vi "FipsAdjacent.vi"() -> (11 "Fips":i32[](array[numeric]))   [LabVIEW 2017] (continued)
\"Lake County, FL\"\t12069\n\"Volusia County, FL\"\t12127\t\"Marion County, FL\"\t12083\n\"Volusia County, FL\"\t12127\t\"Orange County, FL\"\t12095\n\"Volusia County, FL\"\t12127\t\"Putnam County, FL\"\t12107\n\"Volusia County, FL\"\t12127\t\"Seminole County, FL\"\t12117\n\"Volusia County, FL\"\t12127\t\"Volusia County, FL\"\t12127\n\"Wakulla County, FL\"\t12129\t\"Franklin County, FL\"\t12037\n\"Wakulla County, FL\"\t12129\t\"Jefferson County, FL\"\t12065\n\"Wakulla County, FL\"\t12129\t\"Leon County, FL\"\t12073\n\"Wakulla County, FL\"\t12129\t\"Liberty County, FL\"\t12077\n\"Wakulla County, FL\"\t12129\t\"Wakulla County, FL\"\t12129\n\"Walton County, FL\"\t12131\t\"Covington County, AL\"\t01039\n\"Walton County, FL\"\t12131\t\"Geneva County, AL\"\t01061\n\"Walton County, FL\"\t12131\t\"Bay County, FL\"\t12005\n\"Walton County, FL\"\t12131\t\"Holmes County, FL\"\t12059\n\"Walton County, FL\"\t12131\t\"Okaloosa County, FL\"\t12091\n\"Walton County, FL\"\t12131\t\"Walton County, FL\"\t12131\n\"Walton County, FL\"\t12131\t\"Washington County, FL\"\t12133\n\"Washington County, FL\"\t12133\t\"Bay County, FL\"\t12005\n\"Washington County, FL\"\t12133\t\"Holmes County, FL\"\t12059\n\"Washington County, FL\"\t12133\t\"Jackson County, FL\"\t12063\n\"Washington County, FL\"\t12133\t\"Walton County, FL\"\t12131\n\"Washington County, FL\"\t12133\t\"Washington County, FL\"\t12133\n\"Appling County, GA\"\t13001\t\"Appling County, GA\"\t13001\n\"Appling County, GA\"\t13001\t\"Bacon County, GA\"\t13005\n\"Appling County, GA\"\t13001\t\"Jeff Davis County, GA\"\t13161\n\"Appling County, GA\"\t13001\t\"Pierce County, GA\"\t13229\n\"Appling County, GA\"\t13001\t\"Tattnall County, GA\"\t13267\n\"Appling County, GA\"\t13001\t\"Toombs County, GA\"\t13279\n\"Appling County, GA\"\t13001\t\"Wayne County, GA\"\t13305\n\"Atkinson County, GA\"\t13003\t\"Atkinson County, GA\"\t13003\n\"Atkinson County, GA\"\t13003\t\"Berrien County, GA\"\t13019\n\"Atkinson County, GA\"\t13003\t\"Clinch County, GA\"\t13065\n\"Atkinson County, GA\"\t13003\t\"Coffee County, GA\"\t13069\n\"Atkinson County, GA\"\t13003\t\"Lanier County, GA\"\t13173\n\"Atkinson County, GA\"\t13003\t\"Ware County, GA\"\t13299\n\"Bacon County, GA\"\t13005\t\"Appling County, GA\"\t13001\n\"Bacon County, GA\"\t13005\t\"Bacon County, GA\"\t13005\n\"Bacon County, GA\"\t13005\t\"Coffee County, GA\"\t13069\n\"Bacon County, GA\"\t13005\t\"Jeff Davis County, GA\"\t13161\n\"Bacon County, GA\"\t13005\t\"Pierce County, GA\"\t13229\n\"Bacon County, GA\"\t13005\t\"Ware County, GA\"\t13299\n\"Baker County, GA\"\t13007\t\"Baker County, GA\"\t13007\n\"Baker County, GA\"\t13007\t\"Calhoun County, GA\"\t13037\n\"Baker County, GA\"\t13007\t\"Decatur County, GA\"\t13087\n\"Baker County, GA\"\t13007\t\"Dougherty County, GA\"\t13095\n\"Baker County, GA\"\t13007\t\"Early County, GA\"\t13099\n\"Baker County, GA\"\t13007\t\"Miller County, GA\"\t13201\n\"Baker County, GA\"\t13007\t\"Mitchell County, GA\"\t13205\n\"Baldwin County, GA\"\t13009\t\"Baldwin County, GA\"\t13009\n\"Baldwin County, GA\"\t13009\t\"Hancock County, GA\"\t13141\n\"Baldwin County, GA\"\t13009\t\"Jones County, GA\"\t13169\n\"Baldwin County, GA\"\t13009\t\"Putnam County, GA\"\t13237\n\"Baldwin County, GA\"\t13009\t\"Washington County, GA\"\t13303\n\"Baldwin County, GA\"\t13009\t\"Wilkinson County, GA\"\t13319\n\"Banks County, GA\"\t13011\t\"Banks County, GA\"\t13011\n\"Banks County, GA\"\t13011\t\"Franklin County, GA\"\t13119\n\"Banks County, GA\"\t13011\t\"Habersham County, GA\"\t13137\n\"Banks County, GA\"\t13011\t\"Hall County, GA\"\t13139\n\"Banks County, GA\"\t13011\t\"Jackson County, GA\"\t13157\n\"Banks County, GA\"\t13011\t\"Madison County, GA\"\t13195\n\"Banks County, GA\"\t13011\t\"Stephens County, GA\"\t13257\n\"Barrow County, GA\"\t13013\t\"Barrow County, GA\"\t13013\n\"Barrow County, GA\"\t13013\t\"Clarke County, GA\"\t13059\n\"Barrow County, GA\"\t13013\t\"Gwinnett County, GA\"\t13135\n\"Barrow County, GA\"\t13013\t\"Hall County, GA\"\t13139\n\"Barrow County, GA\"\t13013\t\"Jackson County, GA\"\t13157\n\"Barrow County, GA\"\t13013\t\"Oconee County, GA\"\t13219\n\"Barrow County, GA\"\t13013\t\"Walton County, GA\"\t13297\n\"Bartow County, GA\"\t13015\t\"Bartow County, GA\"\t13015\n\"Bartow County, GA\"\t13015\t\"Cherokee County, GA\"\t13057\n\"Bartow County, GA\"\t13015\t\"Cobb County, GA\"\t13067\n\"Bartow County, GA\"\t13015\t\"Floyd County, GA\"\t13115\n\"Bartow County, GA\"\t13015\t\"Gordon County, GA\"\t13129\n\"Bartow County, GA\"\t13015\t\"Paulding County, GA\"\t13223\n\"Bartow County, GA\"\t13015\t\"Pickens County, GA\"\t13227\n\"Bartow County, GA\"\t13015\t\"Polk County, GA\"\t13233\n\"Ben Hill County, GA\"\t13017\t\"Ben Hill County, GA\"\t13017\n\"Ben Hill County, GA\"\t13017\t\"Coffee County, GA\"\t13069\n\"Ben Hill County, GA\"\t13017\t\"Irwin County, GA\"\t13155\n\"Ben Hill County, GA\"\t13017\t\"Telfair County, GA\"\t13271\n\"Ben Hill County, GA\"\t13017\t\"Turner County, GA\"\t13287\n\"Ben Hill County, GA\"\t13017\t\"Wilcox County, GA\"\t13315\n\"Berrien County, GA\"\t13019\t\"Atkinson County, GA\"\t13003\n\"Berrien County, GA\"\t13019\t\"Berrien County, GA\"\t13019\n\"Berrien County, GA\"\t13019\t\"Coffee County, GA\"\t13069\n\"Berrien County, GA\"\t13019\t\"Cook County, GA\"\t13075\n\"Berrien County, GA\"\t13019\t\"Irwin County, GA\"\t13155\n\"Berrien County, GA\"\t13019\t\"Lanier County, GA\"\t13173\n\"Berrien County, GA\"\t13019\t\"Lowndes County, GA\"\t13185\n\"Berrien County, GA\"\t13019\t\"Tift County, GA\"\t13277\n\"Bibb County, GA\"\t13021\t\"Bibb County, GA\"\t13021\n\"Bibb County, GA\"\t13021\t\"Crawford County, GA\"\t13079\n\"Bibb County, GA\"\t13021\t\"Houston County, GA\"\t13153\n\"Bibb County, GA\"\t13021\t\"Jones County, GA\"\t13169\n\"Bibb County, GA\"\t13021\t\"Monroe County, GA\"\t13207\n\"Bibb County, GA\"\t13021\t\"Twiggs County, GA\"\t13289\n\"Bleckley County, GA\"\t13023\t\"Bleckley County, GA\"\t13023\n\"Bleckley County, GA\"\t13023\t\"Dodge County, GA\"\t13091\n\"Bleckley County, GA\"\t13023\t\"Houston County, GA\"\t13153\n\"Bleckley County, GA\"\t13023\t\"Laurens County, GA\"\t13175\n\"Bleckley County, GA\"\t13023\t\"Pulaski County, GA\"\t13235\n\"Bleckley County, GA\"\t13023\t\"Twiggs County, GA\"\t13289\n\"Bleckley County, GA\"\t13023\t\"Wilkinson County, GA\"\t13319\n\"Brantley County, GA\"\t13025\t\"Brantley County, GA\"\t13025\n\"Brantley County, GA\"\t13025\t\"Camden County, GA\"\t13039\n\"Brantley County, GA\"\t13025\t\"Charlton County, GA\"\t13049\n\"Brantley County, GA\"\t13025\t\"Glynn County, GA\"\t13127\n\"Brantley County, GA\"\t13025\t\"Pierce County, GA\"\t13229\n\"Brantley County, GA\"\t13025\t\"Ware County, GA\"\t13299\n\"Brantley County, GA\"\t13025\t\"Wayne County, GA\"\t13305\n\"Brooks County, GA\"\t13027\t\"Hamilton County, FL\"\t12047\n\"Brooks County, GA\"\t13027\t\"Jefferson County, FL\"\t12065\n\"Brooks County, GA\"\t13027\t\"Madison County, FL\"\t12079\n\"Brooks County, GA\"\t13027\t\"Brooks County, GA\"\t13027\n\"Brooks County, GA\"\t13027\t\"Colquitt County, GA\"\t13071\n\"Brooks County, GA\"\t13027\t\"Cook County, GA\"\t13075\n\"Brooks County, GA\"\t13027\t\"Lowndes County, GA\"\t13185\n\"Brooks County, GA\"\t13027\t\"Thomas County, GA\"\t13275\n\"Bryan County, GA\"\t13029\t\"Bryan County, GA\"\t13029\n\"Bryan County, GA\"\t13029\t\"Bulloch County, GA\"\t13031\n\"Bryan County, GA\"\t13029\t\"Chatham County, GA\"\t13051\n\"Bryan County, GA\"\t13029\t\"Effingham County, GA\"\t13103\n\"Bryan County, GA\"\t13029\t\"Evans County, GA\"\t13109\n\"Bryan County, GA\"\t13029\t\"Liberty County, GA\"\t13179\n\"Bulloch County, GA\"\t13031\t\"Bryan County, GA\"\t13029\n\"Bulloch County, GA\"\t13031\t\"Bulloch County, GA\"\t13031\n\"Bulloch County, GA\"\t13031\t\"Candler County, GA\"\t13043\n\"Bulloch County, GA\"\t13031\t\"Effingham County, GA\"\t13103\n\"Bulloch County, GA\"\t13031\t\"Emanuel County, GA\"\t13107\n\"Bulloch County, GA\"\t13031\t\"Evans County, GA\"\t13109\n\"Bulloch County, GA\"\t13031\t\"Jenkins County, GA\"\t13165\n\"Bulloch County, GA\"\t13031\t\"Screven County, GA\"\t13251\n\"Burke County, GA\"\t13033\t\"Burke County, GA\"\t13033\n\"Burke County, GA\"\t13033\t\"Emanuel County, GA\"\t13107\n\"Burke County, GA\"\t13033\t\"Jefferson County, GA\"\t13163\n\"Burke County, GA\"\t13033\t\"Jenkins County, GA\"\t13165\n\"Burke County, GA\"\t13033\t\"Richmond County, GA\"\t13245\n\"Burke County, GA\"\t13033\t\"Screven County, GA\"\t13251\n\"Burke County, GA\"\t13033\t\"Aiken County, SC\"\t45003\n\"Burke County, GA\"\t13033\t\"Allendale County, SC\"\t45005\n\"Burke County, GA\"\t13033\t\"Barnwell County, SC\"\t45011\n\"Butts County, GA\"\t13035\t\"Butts County, GA\"\t13035\n\"Butts County, GA\"\t13035\t\"Henry County, GA\"\t13151\n\"Butts County, GA\"\t13035\t\"Jasper County, GA\"\t13159\n\"Butts County, GA\"\t13035\t\"Lamar County, GA\"\t13171\n\"Butts County, GA\"\t13035\t\"Monroe County, GA\"\t13207\n\"Butts County, GA\"\t13035\t\"Newton County, GA\"\t13217\n\"Butts County, GA\"\t13035\t\"Spalding County, GA\"\t13255\n\"Calhoun County, GA\"\t13037\t\"Baker County, GA\"\t13007\n\"Calhoun County, GA\"\t13037\t\"Calhoun County, GA\"\t13037\n\"Calhoun County, GA\"\t13037\t\"Clay County, GA\"\t13061\n\"Calhoun County, GA\"\t13037\t\"Dougherty County, GA\"\t13095\n\"Calhoun County, GA\"\t13037\t\"Early County, GA\"\t13099\n\"Calhoun County, GA\"\t13037\t\"Randolph County, GA\"\t13243\n\"Calhoun County, GA\"\t13037\t\"Terrell County, GA\"\t13273\n\"Camden County, GA\"\t13039\t\"Nassau County, FL\"\t12089\n\"Camden County, GA\"\t13039\t\"Brantley County, GA\"\t13025\n\"Camden County, GA\"\t13039\t\"Camden County, GA\"\t13039\n\"Camden County, GA\"\t13039\t\"Charlton County, GA\"\t13049\n\"Camden County, GA\"\t13039\t\"Glynn County, GA\"\t13127\n\"Candler County, GA\"\t13043\t\"Bulloch County, GA\"\t13031\n\"Candler County, GA\"\t13043\t\"Candler County, GA\"\t13043\n\"Candler County, GA\"\t13043\t\"Emanuel County, GA\"\t13107\n\"Candler County, GA\"\t13043\t\"Evans County, GA\"\t13109\n\"Candler County, GA\"\t13043\t\"Tattnall County, GA\"\t13267\n\"Candler County, GA\"\t13043\t\"Toombs County, GA\"\t13279\n\"Carroll County, GA\"\t13045\t\"Cleburne County, AL\"\t01029\n\"Carroll County, GA\"\t13045\t\"Randolph County, AL\"\t01111\n\"Carroll County, GA\"\t13045\t\"Carroll County, GA\"\t13045\n\"Carroll County, GA\"\t13045\t\"Coweta County, GA\"\t13077\n\"Carroll County, GA\"\t13045\t\"Douglas County, GA\"\t13097\n\"Carroll County, GA\"\t13045\t\"Fulton County, GA\"\t13121\n\"Carroll County, GA\"\t13045\t\"Haralson County, GA\"\t13143\n\"Carroll County, GA\"\t13045\t\"Heard County, GA\"\t13149\n\"Carroll County, GA\"\t13045\t\"Paulding County, GA\"\t13223\n\"Catoosa County, GA\"\t13047\t\"Catoosa County, GA\"\t13047\n\"Catoosa County, GA\"\t13047\t\"Walker County, GA\"\t13295\n\"Catoosa County, GA\"\t13047\t\"Whitfield County, GA\"\t13313\n\"Catoosa County, GA\"\t13047\t\"Hamilton County, TN\"\t47065\n\"Charlton County, GA\"\t13049\t\"Baker County, FL\"\t12003\n\"Charlton County, GA\"\t13049\t\"Nassau County, FL\"\t12089\n\"Charlton County, GA\"\t13049\t\"Brantley County, GA\"\t13025\n\"Charlton County, GA\"\t13049\t\"Camden County, GA\"\t13039\n\"Charlton County, GA\"\t13049\t\"Charlton County, GA\"\t13049\n\"Charlton County, GA\"\t13049\t\"Ware County, GA\"\t13299\n\"Chatham County, GA\"\t13051\t\"Bryan County, GA\"\t13029\n\"Chatham County, GA\"\t13051\t\"Chatham County, GA\"\t13051\n\"Chatham County, GA\"\t13051\t\"Effingham County, GA\"\t13103\n\"Chatham County, GA\"\t13051\t\"Liberty County, GA\"\t13179\n\"Chatham County, GA\"\t13051\t\"Jasper County, SC\"\t45053\n\"Chattahoochee County, GA\"\t13053\t\"Russell County, AL\"\t01113\n\"Chattahoochee County, GA\"\t13053\t\"Chattahoochee County, GA\"\t13053\n\"Chattahoochee County, GA\"\t13053\t\"Marion County, GA\"\t13197\n\"Chattahoochee County, GA\"\t13053\t\"Muscogee County, GA\"\t13215\n\"Chattahoochee County, GA\"\t13053\t\"Stewart County, GA\"\t13259\n\"Chattahoochee County, GA\"\t13053\t\"Talbot County, GA\"\t13263\n\"Chattooga County, GA\"\t13055\t\"Cherokee County, AL\"\t01019\n\"Chattooga County, GA\"\t13055\t\"DeKalb County, AL\"\t01049\n\"Chattooga County, GA\"\t13055\t\"Chattooga County, GA\"\t13055\n\"Chattooga County, GA\"\t13055\t\"Floyd County, GA\"\t13115\n\"Chattooga County, GA\"\t13055\t\"Walker County, GA\"\t13295\n\"Cherokee County, GA\"\t13057\t\"Bartow County, GA\"\t13015\n\"Cherokee County, GA\"\t13057\t\"Cherokee County, GA\"\t13057\n\"Cherokee County, GA\"\t13057\t\"Cobb County, GA\"\t13067\n\"Cherokee County, GA\"\t13057\t\"Dawson County, GA\"\t13085\n\"Cherokee County, GA\"\t13057\t\"Forsyth County, GA\"\t13117\n\"Cherokee County, GA\"\t13057\t\"Fulton County, GA\"\t13121\n\"Cherokee County, GA\"\t13057\t\"Gordon County, GA\"\t13129\n\"Cherokee County, GA\"\t13057\t\"Pickens County, GA\"\t13227\n\"Clarke County, GA\"\t13059\t\"Barrow County, GA\"\t13013\n\"Clarke County, GA\"\t13059\t\"Clarke County, GA\"\t13059\n\"Clarke County, GA\"\t13059\t\"Jackson County, GA\"\t13157\n\"Clarke County, GA\"\t13059\t\"Madison County, GA\"\t13195\n\"Clarke County, GA\"\t13059\t\"Oconee County, GA\"\t13219\n\"Clarke County, GA\"\t13059\t\"Oglethorpe County, GA\"\t13221\n\"Clay County, GA\"\t13061\t\"Barbour County, AL\"\t01005\n\"Clay County, GA\"\t13061\t\"Henry County, AL\"\t01067\n\"Clay County, GA\"\t13061\t\"Calhoun County, GA\"\t13037\n\"Clay County, GA\"\t13061\t\"Clay County, GA\"\t13061\n\"Clay County, GA\"\t13061\t\"Early County, GA\"\t13099\n\"Clay County, GA\"\t13061\t\"Quitman County, GA\"\t13239\n\"Clay County, GA\"\t13061\t\"Randolph County, GA\"\t13243\n\"Clayton County, GA\"\t13063\t\"Clayton County, GA\"\t13063\n\"Clayton County, GA\"\t13063\t\"DeKalb County, GA\"\t13089\n\"Clayton County, GA\"\t13063\t\"Fayette County, GA\"\t13113\n\"Clayton County, GA\"\t13063\t\"Fulton County, GA\"\t13121\n\"Clayton County, GA\"\t13063\t\"Henry County, GA\"\t13151\n\"Clayton County, GA\"\t13063\t\"Spalding County, GA\"\t13255\n\"Clinch County, GA\"\t13065\t\"Baker County, FL\"\t12003\n\"Clinch County, GA\"\t13065\t\"Columbia County, FL\"\t12023\n\"Clinch County, GA\"\t13065\t\"Atkinson County, GA\"\t13003\n\"Clinch County, GA\"\t13065\t\"Clinch County, GA\"\t13065\n\"Clinch County, GA\"\t13065\t\"Echols County, GA\"\t13101\n\"Clinch County, GA\"\t13065\t\"Lanier County, GA\"\t13173\n\"Clinch County, GA\"\t13065\t\"Ware County, GA\"\t13299\n\"Cobb County, GA\"\t13067\t\"Bartow County, GA\"\t13015\n\"Cobb County, GA\"\t13067\t\"Cherokee County, GA\"\t13057\n\"Cobb County, GA\"\t13067\t\"Cobb County, GA\"\t13067\n\"Cobb County, GA\"\t13067\t\"Douglas County, GA\"\t13097\n\"Cobb County, GA\"\t13067\t\"Fulton County, GA\"\t13121\n\"Cobb County, GA\"\t13067\t\"Paulding County, GA\"\t13223\n\"Coffee County, GA\"\t13069\t\"Atkinson County, GA\"\t13003\n\"Coffee County, GA\"\t13069\t\"Bacon County, GA\"\t13005\n\"Coffee County, GA\"\t13069\t\"Ben Hill County, GA\"\t13017\n\"Coffee County, GA\"\t13069\t\"Berrien County, GA\"\t13019\n\"Coffee County, GA\"\t13069\t\"Coffee County, GA\"\t13069\n\"Coffee County, GA\"\t13069\t\"Irwin County, GA\"\t13155\n\"Coffee County, GA\"\t13069\t\"Jeff Davis County, GA\"\t13161\n\"Coffee County, GA\"\t13069\t\"Telfair County, GA\"\t13271\n\"Coffee County, GA\"\t13069\t\"Ware County, GA\"\t13299\n\"Colquitt County, GA\"\t13071\t\"Brooks County, GA\"\t13027\n\"Colquitt County, GA\"\t13071\t\"Colquitt County, GA\"\t13071\n\"Colquitt County, GA\"\t13071\t\"Cook County, GA\"\t13075\n\"Colquitt County, GA\"\t13071\t\"Mitchell County, GA\"\t13205\n\"Colquitt County, GA\"\t13071\t\"Thomas County, GA\"\t13275\n\"Colquitt County, GA\"\t13071\t\"Tift County, GA\"\t13277\n\"Colquitt County, GA\"\t13071\t\"Worth County, GA\"\t13321\n\"Columbia County, GA\"\t13073\t\"Columbia County, GA\"\t13073\n\"Columbia County, GA\"\t13073\t\"Lincoln County, GA\"\t13181\n\"Columbia County, GA\"\t13073\t\"McDuffie County, GA\"\t13189\n\"Columbia County, GA\"\t13073\t\"Richmond County, GA\"\t13245\n\"Columbia County, GA\"\t13073\t\"Edgefield County, SC\"\t45037\n\"Columbia County, GA\"\t13073\t\"McCormick County, SC\"\t45065\n\"Cook County, GA\"\t13075\t\"Berrien County, GA\"\t13019\n\"Cook County, GA\"\t13075\t\"Brooks County, GA\"\t13027\n\"Cook County, GA\"\t13075\t\"Colquitt County, GA\"\t13071\n\"Cook County, GA\"\t13075\t\"Cook County, GA\"\t13075\n\"Cook County, GA\"\t13075\t\"Lowndes County, GA\"\t13185\n\"Cook County, GA\"\t13075\t\"Tift County, GA\"\t13277\n\"Coweta County, GA\"\t13077\t\"Carroll County, GA\"\t13045\n\"Coweta County, GA\"\t13077\t\"Coweta County, GA\"\t13077\n\"Coweta County, GA\"\t13077\t\"Fayette County, GA\"\t13113\n\"Coweta County, GA\"\t13077\t\"Fulton County, GA\"\t13121\n\"Coweta County, GA\"\t13077\t\"Heard County, GA\"\t13149\n\"Coweta County, GA\"\t13077\t\"Meriwether County, GA\"\t13199\n\"Coweta County, GA\"\t13077\t\"Spalding County, GA\"\t13255\n\"Coweta County, GA\"\t13077\t\"Troup County, GA\"\t13285\n\"Crawford County, GA\"\t13079\t\"Bibb County, GA\"\t13021\n\"Crawford County, GA\"\t13079\t\"Crawford County, GA\"\t13079\n\"Crawford County, GA\"\t13079\t\"Houston County, GA\"\t13153\n\"Crawford County, GA\"\t13079\t\"Macon County, GA\"\t13193\n\"Crawford County, GA\"\t13079\t\"Monroe County, GA\"\t13207\n\"Crawford County, GA\"\t13079\t\"Peach County, GA\"\t13225\n\"Crawford County, GA\"\t13079\t\"Taylor County, GA\"\t13269\n\"Crawford County, GA\"\t13079\t\"Upson County, GA\"\t13293\n\"Crisp County, GA\"\t13081\t\"Crisp County, GA\"\t13081\n\"Crisp County, GA\"\t13081\t\"Dooly County, GA\"\t13093\n\"Crisp County, GA\"\t13081\t\"Lee County, GA\"\t13177\n\"Crisp County, GA\"\t13081\t\"Sumter County, GA\"\t13261\n\"Crisp County, GA\"\t13081\t\"Turner County, GA\"\t13287\n\"Crisp County, GA\"\t13081\t\"Wilcox County, GA\"\t13315\n\"Crisp County, GA\"\t13081\t\"Worth County, GA\"\t13321\n\"Dade County, GA\"\t13083\t\"DeKalb County, AL\"\t01049\n\"Dade County, GA\"\t13083\t\"Jackson County, AL\"\t01071\n\"Dade County, GA\"\t13083\t\"Dade County, GA\"\t13083\n\"Dade County, GA\"\t13083\t\"Walker County, GA\"\t13295\n\"Dade County, GA\"\t13083\t\"Hamilton County, TN\"\t47065\n\"Dade County, GA\"\t13083\t\"Marion County, TN\"\t47115\n\"Dawson County, GA\"\t13085\t\"Cherokee County, GA\"\t13057\n\"Dawson County, GA\"\t13085\t\"Dawson County, GA\"\t13085\n\"Dawson County, GA\"\t13085\t\"Fannin County, GA\"\t13111\n\"Dawson County, GA\"\t13085\t\"Forsyth County, GA\"\t13117\n\"Dawson County, GA\"\t13085\t\"Gilmer County, GA\"\t13123\n\"Dawson County, GA\"\t13085\t\"Hall County, GA\"\t13139\n\"Dawson County, GA\"\t13085\t\"Lumpkin County, GA\"\t13187\n\"Dawson County, GA\"\t13085\t\"Pickens County, GA\"\t13227\n\"Decatur County, GA\"\t13087\t\"Gadsden County, FL\"\t12039\n\"Decatur County, GA\"\t13087\t\"Baker County, GA\"\t13007\n\"Decatur County, GA\"\t13087\t\"Decatur County, GA\"\t13087\n\"Decatur County, GA\"\t13087\t\"Grady County, GA\"\t13131\n\"Decatur County, GA\"\t13087\t\"Miller County, GA\"\t13201\n\"Decatur County, GA\"\t13087\t\"Mitchell County, GA\"\t13205\n\"Decatur County, GA\"\t13087\t\"Seminole County, GA\"\t13253\n\"DeKalb County, GA\"\t13089\t\"Clayton County, GA\"\t13063\n\"DeKalb County, GA\"\t13089\t\"DeKalb County, GA\"\t13089\n\"DeKalb County, GA\"\t13089\t\"Fulton County, GA\"\t13121\n\"DeKalb County, GA\"\t13089\t\"Gwinnett County, GA\"\t13135\n\"DeKalb County, GA\"\t13089\t\"Henry County, GA\"\t13151\n\"DeKalb County, GA\"\t13089\t\"Rockdale County, GA\"\t13247\n\"Dodge County, GA\"\t13091\t\"Bleckley County, GA\"\t13023\n\"Dodge County, GA\"\t13091\t\"Dodge County, GA\"\t13091\n\"Dodge County, GA\"\t13091\t\"Laurens County, GA\"\t13175\n\"Dodge County, GA\"\t13091\t\"Pulaski County, GA\"\t13235\n\"Dodge County, GA\"\t13091\t\"Telfair County, GA\"\t13271\n\"Dodge County, GA\"\t13091\t\"Wheeler County, GA\"\t13309\n\"Dodge County, GA\"\t13091\t\"Wilcox County, GA\"\t13315\n\"Dooly County, GA\"\t13093\t\"Crisp County, GA\"\t13081\n\"Dooly County, GA\"\t13093\t\"Dooly County, GA\"\t13093\n\"Dooly County, GA\"\t13093\t\"Houston County, GA\"\t13153\n\"Dooly County, GA\"\t13093\t\"Macon County, GA\"\t13193\n\"Dooly County, GA\"\t13093\t\"Pulaski County, GA\"\t13235\n\"Dooly County, GA\"\t13093\t\"Sumter County, GA\"\t13261\n\"Dooly County, GA\"\t13093\t\"Wilcox County, GA\"\t13315\n\"Dougherty County, GA\"\t13095\t\"Baker County, GA\"\t13007\n\"Dougherty County, GA\"\t13095\t\"Calhoun County, GA\"\t13037\n\"Dougherty County, GA\"\t13095\t\"Dougherty County, GA\"\t13095\n\"Dougherty County, GA\"\t13095\t\"Lee County, GA\"\t13177\n\"Dougherty County, GA\"\t13095\t\"Mitchell County, GA\"\t13205\n\"Dougherty County, GA\"\t13095\t\"Terrell County, GA\"\t13273\n\"Dougherty County, GA\"\t13095\t\"Worth County, GA\"\t13321\n\"Douglas County, GA\"\t13097\t\"Carroll County, GA\"\t13045\n\"Douglas County, GA\"\t13097\t\"Cobb County, GA\"\t13067\n\"Douglas County, GA\"\t13097\t\"Douglas County, GA\"\t13097\n\"Douglas County, GA\"\t13097\t\"Fulton County, GA\"\t13121\n\"Douglas County, GA\"\t13097\t\"Paulding County, GA\"\t13223\n\"Early County, GA\"\t13099\t\"Henry County, AL\"\t01067\n\"Early County, GA\"\t13099\t\"Houston County, AL\"\t01069\n\"Early County, GA\"\t13099\t\"Baker County, GA\"\t13007\n\"Early County, GA\"\t13099\t\"Calhoun County, GA\"\t13037\n\"Early County, GA\"\t13099\t\"Clay County, GA\"\t13061\n\"Early County, GA\"\t13099\t\"Early County, GA\"\t13099\n\"Early County, GA\"\t13099\t\"Miller County, GA\"\t13201\n\"Early County, GA\"\t13099\t\"Seminole County, GA\"\t13253\n\"Echols County, GA\"\t13101\t\"Columbia County, FL\"\t12023\n\"Echols County, GA\"\t13101\t\"Hamilton County, FL\"\t12047\n\"Echols County, GA\"\t13101\t\"Clinch County, GA\"\t13065\n\"Echols County, GA\"\t13101\t\"Echols County, GA\"\t13101\n\"Echols County, GA\"\t13101\t\"Lanier County, GA\"\t13173\n\"Echols County, GA\"\t13101\t\"Lowndes County, GA\"\t13185\n\"Effingham County, GA\"\t13103\t\"Bryan County, GA\"\t13029\n\"Effingham County, GA\"\t13103\t\"Bulloch County, GA\"\t13031\n\"Effingham County, GA\"\t13103\t\"Chatham County, GA\"\t13051\n\"Effingham County, GA\"\t13103\t\"Effingham County, GA\"\t13103\n\"Effingham County, GA\"\t13103\t\"Screven County, GA\"\t13251\n\"Effingham County, GA\"\t13103\t\"Hampton County, SC\"\t45049\n\"Effingham County, GA\"\t13103\t\"Jasper County, SC\"\t45053\n\"Elbert County, GA\"\t13105\t\"Elbert County, GA\"\t13105\n\"Elbert County, GA\"\t13105\t\"Hart County, GA\"\t13147\n\"Elbert County, GA\"\t13105\t\"Lincoln County, GA\"\t13181\n\"Elbert County, GA\"\t13105\t\"Madison County, GA\"\t13195\n\"Elbert County, GA\"\t13105\t\"Oglethorpe County, GA\"\t13221\n\"Elbert County, GA\"\t13105\t\"Wilkes County, GA\"\t13317\n\"Elbert County, GA\"\t13105\t\"Abbeville County, SC\"\t45001\n\"Elbert County, GA\"\t13105\t\"Anderson County, SC\"\t45007\n\"Elbert County, GA\"\t13105\t\"McCormick County, SC\"\t45065\n\"Emanuel County, GA\"\t13107\t\"Bulloch County, GA\"\t13031\n\"Emanuel County, GA\"\t13107\t\"Burke County, GA\"\t13033\n\"Emanuel County, GA\"\t13107\t\"Candler County, GA\"\t13043\n\"Emanuel County, GA\"\t13107\t\"Emanuel County, GA\"\t13107\n\"Emanuel County, GA\"\t13107\t\"Jefferson County, GA\"\t13163\n\"Emanuel County, GA\"\t13107\t\"Jenkins County, GA\"\t13165\n\"Emanuel County, GA\"\t13107\t\"Johnson County, GA\"\t13167\n\"Emanuel County, GA\"\t13107\t\"Laurens County, GA\"\t13175\n\"Emanuel County, GA\"\t13107\t\"Tattnall County, GA\"\t13267\n\"Emanuel County, GA\"\t13107\t\"Toombs County, GA\"\t13279\n\"Emanuel County, GA\"\t13107\t\"Treutlen County, GA\"\t13283\n\"Evans County, GA\"\t13109\t\"Bryan County, GA\"\t13029\n\"Evans County, GA\"\t13109\t\"Bulloch County, GA\"\t13031\n\"Evans County, GA\"\t13109\t\"Candler County, GA\"\t13043\n\"Evans County, GA\"\t13109\t\"Evans County, GA\"\t13109\n\"Evans County, GA\"\t13109\t\"Liberty County, GA\"\t13179\n\"Evans County, GA\"\t13109\t\"Tattnall County, GA\"\t13267\n\"Fannin County, GA\"\t13111\t\"Dawson County, GA\"\t13085\n\"Fannin County, GA\"\t13111\t\"Fannin County, GA\"\t13111\n\"Fannin County, GA\"\t13111\t\"Gilmer County, GA\"\t13123\n\"Fannin County, GA\"\t13111\t\"Lumpkin County, GA\"\t13187\n\"Fannin County, GA\"\t13111\t\"Murray County, GA\"\t13213\n\"Fannin County, GA\"\t13111\t\"Union County, GA\"\t13291\n\"Fannin County, GA\"\t13111\t\"Cherokee County, NC\"\t37039\n\"Fannin County, GA\"\t13111\t\"Polk County, TN\"\t47139\n\"Fayette County, GA\"\t13113\t\"Clayton County, GA\"\t13063\n\"Fayette County, GA\"\t13113\t\"Coweta County, GA\"\t13077\n\"Fayette County, GA\"\t13113\t\"Fayette County, GA\"\t13113\n\"Fayette County, GA\"\t13113\t\"Fulton County, GA\"\t13121\n\"Fayette County, GA\"\t13113\t\"Spalding County, GA\"\t13255\n\"Floyd County, GA\"\t13115\t\"Cherokee County, AL\"\t01019\n\"Floyd County, GA\"\t13115\t\"Bartow County, GA\"\t13015\n\"Floyd County, GA\"\t13115\t\"Chattooga County, GA\"\t13055\n\"Floyd County, GA\"\t13115\t\"Floyd County, GA\"\t13115\n\"Floyd County, GA\"\t13115\t\"Gordon County, GA\"\t13129\n\"Floyd County, GA\"\t13115\t\"Polk County, GA\"\t13233\n\"Floyd County, GA\"\t13115\t\"Walker County, GA\"\t13295\n\"Forsyth County, GA\"\t13117\t\"Cherokee County, GA\"\t13057\n\"Forsyth County, GA\"\t13117\t\"Dawson County, GA\"\t13085\n\"Forsyth County, GA\"\t13117\t\"Forsyth County, GA\"\t13117\n\"Forsyth County, GA\"\t13117\t\"Fulton County, GA\"\t13121\n\"Forsyth County, GA\"\t13117\t\"Gwinnett County, GA\"\t13135\n\"Forsyth County, GA\"\t13117\t\"Hall County, GA\"\t13139\n\"Franklin County, GA\"\t13119\t\"Banks County, GA\"\t13011\n\"Franklin County, GA\"\t13119\t\"Franklin County, GA\"\t13119\n\"Franklin County, GA\"\t13119\t\"Hart County, GA\"\t13147\n\"Franklin County, GA\"\t13119\t\"Madison County, GA\"\t13195\n\"Franklin County, GA\"\t13119\t\"Stephens County, GA\"\t13257\n\"Franklin County, GA\"\t13119\t\"Oconee County, SC\"\t45073\n\"Fulton County, GA\"\t13121\t\"Carroll County, GA\"\t13045\n\"Fulton County, GA\"\t13121\t\"Cherokee County, GA\"\t13057\n\"Fulton County, GA\"\t13121\t\"Clayton County, GA\"\t13063\n\"Fulton County, GA\"\t13121\t\"Cobb County, GA\"\t13067\n\"Fulton County, GA\"\t13121\t\"Coweta County, GA\"\t13077\n\"Fulton County, GA\"\t13121\t\"DeKalb County, GA\"\t13089\n\"Fulton County, GA\"\t13121\t\"Douglas County, GA\"\t13097\n\"Fulton County, GA\"\t13121\t\"Fayette County, GA\"\t13113\n\"Fulton County, GA\"\t13121\t\"Forsyth County, GA\"\t13117\n\"Fulton County, GA\"\t13121\t\"Fulton County, GA\"\t13121\n\"Fulton County, GA\"\t13121\t\"Gwinnett County, GA\"\t13135\n\"Gilmer County, GA\"\t13123\t\"Dawson County, GA\"\t13085\n\"Gilmer County, GA\"\t13123\t\"Fannin County, GA\"\t13111\n\"Gilmer County, GA\"\t13123\t\"Gilmer County, GA\"\t13123\n\"Gilmer County, GA\"\t13123\t\"Gordon County, GA\"\t13129\n\"Gilmer County, GA\"\t13123\t\"Murray County, GA\"\t13213\n\"Gilmer County, GA\"\t13123\t\"Pickens County, GA\"\t13227\n\"Glascock County, GA\"\t13125\t\"Glascock County, GA\"\t13125\n\"Glascock County, GA\"\t13125\t\"Hancock County, GA\"\t13141\n\"Glascock County, GA\"\t13125\t\"Jefferson County, GA\"\t13163\n\"Glascock County, GA\"\t13125\t\"Warren County, GA\"\t13301\n\"Glascock County, GA\"\t13125\t\"Washington County, GA\"\t13303\n\"Glynn County, GA\"\t13127\t\"Brantley County, GA\"\t13025\n\"Glynn County, GA\"\t13127\t\"Camden County, GA\"\t13039\n\"Glynn County, GA\"\t13127\t\"Glynn County, GA\"\t13127\n\"Glynn County, GA\"\t13127\t\"McIntosh County, GA\"\t13191\n\"Glynn County, GA\"\t13127\t\"Wayne County, GA\"\t13305\n\"Gordon County, GA\"\t13129\t\"Bartow County, GA\"\t13015\n\"Gordon County, GA\"\t13129\t\"Cherokee County, GA\"\t13057\n\"Gordon County, GA\"\t13129\t\"Floyd County, GA\"\t13115\n\"Gordon County, GA\"\t13129\t\"Gilmer County, GA\"\t13123\n\"Gordon County, GA\"\t13129\t\"Gordon County, GA\"\t13129\n\"Gordon County, GA\"\t13129\t\"Murray County, GA\"\t13213\n\"Gordon County, GA\"\t13129\t\"Pickens County, GA\"\t13227\n\"Gordon County, GA\"\t13129\t\"Walker County, GA\"\t13295\n\"Gordon County, GA\"\t13129\t\"Whitfield County, GA\"\t13313\n\"Grady County, GA\"\t13131\t\"Gadsden County, FL\"\t12039\n\"Grady County, GA\"\t13131\t\"Leon County, FL\"\t12073\n\"Grady County, GA\"\t13131\t\"Decatur County, GA\"\t13087\n\"Grady County, GA\"\t13131\t\"Grady County, GA\"\t13131\n\"Grady County, GA\"\t13131\t\"Mitchell County, GA\"\t13205\n\"Grady County, GA\"\t13131\t\"Thomas County, GA\"\t13275\n\"Greene County, GA\"\t13133\t\"Greene County, GA\"\t13133\n\"Greene County, GA\"\t13133\t\"Hancock County, GA\"\t13141\n\"Greene County, GA\"\t13133\t\"Morgan County, GA\"\t13211\n\"Greene County, GA\"\t13133\t\"Oconee County, GA\"\t13219\n\"Greene County, GA\"\t13133\t\"Oglethorpe County, GA\"\t13221\n\"Greene County, GA\"\t13133\t\"Putnam County, GA\"\t13237\n\"Greene County, GA\"\t13133\t\"Taliaferro County, GA\"\t13265\n\"Gwinnett County, GA\"\t13135\t\"Barrow County, GA\"\t13013\n\"Gwinnett County, GA\"\t13135\t\"DeKalb County, GA\"\t13089\n\"Gwinnett County, GA\"\t13135\t\"Forsyth County, GA\"\t13117\n\"Gwinnett County, GA\"\t13135\t\"Fulton County, GA\"\t13121\n\"Gwinnett County, GA\"\t13135\t\"Gwinnett County, GA\"\t13135\n\"Gwinnett County, GA\"\t13135\t\"Hall County, GA\"\t13139\n\"Gwinnett County, GA\"\t13135\t\"Jackson County, GA\"\t13157\n\"Gwinnett County, GA\"\t13135\t\"Rockdale County, GA\"\t13247\n\"Gwinnett County, GA\"\t13135\t\"Walton County, GA\"\t13297\n\"Habersham County, GA\"\t13137\t\"Banks County, GA\"\t13011\n\"Habersham County, GA\"\t13137\t\"Habersham County, GA\"\t13137\n\"Habersham County, GA\"\t13137\t\"Hall County, GA\"\t13139\n\"Habersham County, GA\"\t13137\t\"Rabun County, GA\"\t13241\n\"Habersham County, GA\"\t13137\t\"Stephens County, GA\"\t13257\n\"Habersham County, GA\"\t13137\t\"Towns County, GA\"\t13281\n\"Habersham County, GA\"\t13137\t\"White County, GA\"\t13311\n\"Habersham County, GA\"\t13137\t\"Oconee County, SC\"\t45073\n\"Hall County, GA\"\t13139\t\"Banks County, GA\"\t13011\n\"Hall County, GA\"\t13139\t\"Barrow County, GA\"\t13013\n\"Hall County, GA\"\t13139\t\"Dawson County, GA\"\t13085\n\"Hall County, GA\"\t13139\t\"Forsyth County, GA\"\t13117\n\"Hall County, GA\"\t13139\t\"Gwinnett County, GA\"\t13135\n\"Hall County, GA\"\t13139\t\"Habersham County, GA\"\t13137\n\"Hall County, GA\"\t13139\t\"Hall County, GA\"\t13139\n\"Hall County, GA\"\t13139\t\"Jackson County, GA\"\t13157\n\"Hall County, GA\"\t13139\t\"Lumpkin County, GA\"\t13187\n\"Hall County, GA\"\t13139\t\"White County, GA\"\t13311\n\"Hancock County, GA\"\t13141\t\"Baldwin County, GA\"\t13009\n\"Hancock County, GA\"\t13141\t\"Glascock County, GA\"\t13125\n\"Hancock County, GA\"\t13141\t\"Greene County, GA\"\t13133\n\"Hancock County, GA\"\t13141\t\"Hancock County, GA\"\t13141\n\"Hancock County, GA\"\t13141\t\"Putnam County, GA\"\t13237\n\"Hancock County, GA\"\t13141\t\"Taliaferro County, GA\"\t13265\n\"Hancock County, GA\"\t13141\t\"Warren County, GA\"\t13301\n\"Hancock County, GA\"\t13141\t\"Washington County, GA\"\t13303\n\"Haralson County, GA\"\t13143\t\"Cleburne County, AL\"\t01029\n\"Haralson County, GA\"\t13143\t\"Carroll County, GA\"\t13045\n\"Haralson County, GA\"\t13143\t\"Haralson County, GA\"\t13143\n\"Haralson County, GA\"\t13143\t\"Paulding County, GA\"\t13223\n\"Haralson County, GA\"\t13143\t\"Polk County, GA\"\t13233\n\"Harris County, GA\"\t13145\t\"Chambers County, AL\"\t01017\n\"Harris County, GA\"\t13145\t\"Lee County, AL\"\t01081\n\"Harris County, GA\"\t13145\t\"Harris County, GA\"\t13145\n\"Harris County, GA\"\t13145\t\"Meriwether County, GA\"\t13199\n\"Harris County, GA\"\t13145\t\"Muscogee County, GA\"\t13215\n\"Harris County, GA\"\t13145\t\"Talbot County, GA\"\t13263\n\"Harris County, GA\"\t13145\t\"Troup County, GA\"\t13285\n\"Hart County, GA\"\t13147\t\"Elbert County, GA\"\t13105\n\"Hart County, GA\"\t13147\t\"Franklin County, GA\"\t13119\n\"Hart County, GA\"\t13147\t\"Hart County, GA\"\t13147\n\"Hart County, GA\"\t13147\t\"Madison County, GA\"\t13195\n\"Hart County, GA\"\t13147\t\"Anderson County, SC\"\t45007\n\"Hart County, GA\"\t13147\t\"Oconee County, SC\"\t45073\n\"Heard County, GA\"\t13149\t\"Randolph County, AL\"\t01111\n\"Heard County, GA\"\t13149\t\"Carroll County, GA\"\t13045\n\"Heard County, GA\"\t13149\t\"Coweta County, GA\"\t13077\n\"Heard County, GA\"\t13149\t\"Heard County, GA\"\t13149\n\"Heard County, GA\"\t13149\t\"Troup County, GA\"\t13285\n\"Henry County, GA\"\t13151\t\"Butts County, GA\"\t13035\n\"Henry County, GA\"\t13151\t\"Clayton County, GA\"\t13063\n\"Henry County, GA\"\t13151\t\"DeKalb County, GA\"\t13089\n\"Henry County, GA\"\t13151\t\"Henry County, GA\"\t13151\n\"Henry County, GA\"\t13151\t\"Newton County, GA\"\t13217\n\"Henry County, GA\"\t13151\t\"Rockdale County, GA\"\t13247\n\"Henry County, GA\"\t13151\t\"Spalding County, GA\"\t13255\n\"Houston County, GA\"\t13153\t\"Bibb County, GA\"\t13021\n\"Houston County, GA\"\t13153\t\"Bleckley County, GA\"\t13023\n\"Houston County, GA\"\t13153\t\"Crawford County, GA\"\t13079\n\"Houston County, GA\"\t13153\t\"Dooly County, GA\"\t13093\n\"Houston County, GA\"\t13153\t\"Houston County, GA\"\t13153\n\"Houston County, GA\"\t13153\t\"Macon County, GA\"\t13193\n\"Houston County, GA\"\t13153\t\"Peach County, GA\"\t13225\n\"Houston County, GA\"\t13153\t\"Pulaski County, GA\"\t13235\n\"Houston County, GA\"\t13153\t\"Twiggs County, GA\"\t13289\n\"Irwin County, GA\"\t13155\t\"Ben Hill County, GA\"\t13017\n\"Irwin County, GA\"\t13155\t\"Berrien County, GA\"\t13019\n\"Irwin County, GA\"\t13155\t\"Coffee County, GA\"\t13069\n\"Irwin County, GA\"\t13155\t\"Irwin County, GA\"\t13155\n\"Irwin County, GA\"\t13155\t\"Tift County, GA\"\t13277\n\"Irwin County, GA\"\t13155\t\"Turner County, GA\"\t13287\n\"Jackson County, GA\"\t13157\t\"Banks County, GA\"\t13011\n\"Jackson County, GA\"\t13157\t\"Barrow County, GA\"\t13013\n\"Jackson County, GA\"\t13157\t\"Clarke County, GA\"\t13059\n\"Jackson County, GA\"\t13157\t\"Gwinnett County, GA\"\t13135\n\"Jackson County, GA\"\t13157\t\"Hall County, GA\"\t13139\n\"Jackson County, GA\"\t13157\t\"Jackson County, GA\"\t13157\n\"Jackson County, GA\"\t13157\t\"Madison County, GA\"\t13195\n\"Jackson County, GA\"\t13157\t\"Oconee County, GA\"\t13219\n\"Jasper County, GA\"\t13159\t\"Butts County, GA\"\t13035\n\"Jasper County, GA\"\t13159\t\"Jasper County, GA\"\t13159\n\"Jasper County, GA\"\t13159\t\"Jones County, GA\"\t13169\n\"Jasper County, GA\"\t13159\t\"Monroe County, GA\"\t13207\n\"Jasper County, GA\"\t13159\t\"Morgan County, GA\"\t13211\n\"Jasper County, GA\"\t13159\t\"Newton County, GA\"\t13217\n\"Jasper County, GA\"\t13159\t\"Putnam County, GA\"\t13237\n\"Jeff Davis County, GA\"\t13161\t\"Appling County, GA\"\t13001\n\"Jeff Davis County, GA\"\t13161\t\"Bacon County, GA\"\t13005\n\"Jeff Davis County, GA\"\t13161\t\"Coffee County, GA\"\t13069\n\"Jeff Davis County, GA\"\t13161\t\"Jeff Davis County, GA\"\t13161\n\"Jeff Davis County, GA\"\t13161\t\"Montgomery County, GA\"\t13209\n\"Jeff Davis County, GA\"\t13161\t\"Telfair County, GA\"\t13271\n\"Jeff Davis County, GA\"\t13161\t\"Toombs County, GA\"\t13279\n\"Jeff Davis County, GA\"\t13161\t\"Wheeler County, GA\"\t13309\n\"Jefferson County, GA\"\t13163\t\"Burke County, GA\"\t13033\n\"Jefferson County, GA\"\t13163\t\"Emanuel County, GA\"\t13107\n\"Jefferson County, GA\"\t13163\t\"Glascock County, GA\"\t13125\n\"Jefferson County, GA\"\t13163\t\"Jefferson County, GA\"\t13163\n\"Jefferson County, GA\"\t13163\t\"Johnson County, GA\"\t13167\n\"Jefferson County, GA\"\t13163\t\"McDuffie County, GA\"\t13189\n\"Jefferson County, GA\"\t13163\t\"Richmond County, GA\"\t13245\n\"Jefferson County, GA\"\t13163\t\"Warren County, GA\"\t13301\n\"Jefferson County, GA\"\t13163\t\"Washington County, GA\"\t13303\n\"Jenkins County, GA\"\t13165\t\"Bulloch County, GA\"\t13031\n\"Jenkins County, GA\"\t13165\t\"Burke County, GA\"\t13033\n\"Jenkins County, GA\"\t13165\t\"Emanuel County, GA\"\t13107\n\"Jenkins County, GA\"\t13165\t\"Jenkins County, GA\"\t13165\n\"Jenkins County, GA\"\t13165\t\"Screven County, GA\"\t13251\n\"Johnson County, GA\"\t13167\t\"Emanuel County, GA\"\t13107\n\"Johnson County, GA\"\t13167\t\"Jefferson County, GA\"\t13163\n\"Johnson County, GA\"\t13167\t\"Johnson County, GA\"\t13167\n\"Johnson County, GA\"\t13167\t\"Laurens County, GA\"\t13175\n\"Johnson County, GA\"\t13167\t\"Treutlen County, GA\"\t13283\n\"Johnson County, GA\"\t13167\t\"Washington County, GA\"\t13303\n\"Johnson County, GA\"\t13167\t\"Wilkinson County, GA\"\t13319\n\"Jones County, GA\"\t13169\t\"Baldwin County, GA\"\t13009\n\"Jones County, GA\"\t13169\t\"Bibb County, GA\"\t13021\n\"Jones County, GA\"\t13169\t\"Jasper County, GA\"\t13159\n\"Jones County, GA\"\t13169\t\"Jones County, GA\"\t13169\n\"Jones County, GA\"\t13169\t\"Monroe County, GA\"\t13207\n\"Jones County, GA\"\t13169\t\"Putnam County, GA\"\t13237\n\"Jones County, GA\"\t13169\t\"Twiggs County, GA\"\t13289\n\"Jones County, GA\"\t13169\t\"Wilkinson County, GA\"\t13319\n\"Lamar County, GA\"\t13171\t\"Butts County, GA\"\t13035\n\"Lamar County, GA\"\t13171\t\"Lamar County, GA\"\t13171\n\"Lamar County, GA\"\t13171\t\"Monroe County, GA\"\t13207\n\"Lamar County, GA\"\t13171\t\"Pike County, GA\"\t13231\n\"Lamar County, GA\"\t13171\t\"Spalding County, GA\"\t13255\n\"Lamar County, GA\"\t13171\t\"Upson County, GA\"\t13293\n\"Lanier County, GA\"\t13173\t\"Atkinson County, GA\"\t13003\n\"Lanier County, GA\"\t13173\t\"Berrien County, GA\"\t13019\n\"Lanier County, GA\"\t13173\t\"Clinch County, GA\"\t13065\n\"Lanier County, GA\"\t13173\t\"Echols County, GA\"\t13101\n\"Lanier County, GA\"\t13173\t\"Lanier County, GA\"\t13173\n\"Lanier County, GA\"\t13173\t\"Lowndes County, GA\"\t13185\n\"Laurens County, GA\"\t13175\t\"Bleckley County, GA\"\t13023\n\"Laurens County, GA\"\t13175\t\"Dodge County, GA\"\t13091\n\"Laurens County, GA\"\t13175\t\"Emanuel County, GA\"\t13107\n\"Laurens County, GA\"\t13175\t\"Johnson County, GA\"\t13167\n\"Laurens County, GA\"\t13175\t\"Laurens County, GA\"\t13175\n\"Laurens County, GA\"\t13175\t\"Treutlen County, GA\"\t13283\n\"Laurens County, GA\"\t13175\t\"Twiggs County, GA\"\t13289\n\"Laurens County, GA\"\t13175\t\"Wheeler County, GA\"\t13309\n\"Laurens County, GA\"\t13175\t\"Wilkinson County, GA\"\t13319\n\"Lee County, GA\"\t13177\t\"Crisp County, GA\"\t13081\n\"Lee County, GA\"\t13177\t\"Dougherty County, GA\"\t13095\n\"Lee County, GA\"\t13177\t\"Lee County, GA\"\t13177\n\"Lee County, GA\"\t13177\t\"Sumter County, GA\"\t13261\n\"Lee County, GA\"\t13177\t\"Terrell County, GA\"\t13273\n\"Lee County, GA\"\t13177\t\"Worth County, GA\"\t13321\n\"Liberty County, GA\"\t13179\t\"Bryan County, GA\"\t13029\n\"Liberty County, GA\"\t13179\t\"Chatham County, GA\"\t13051\n\"Liberty County, GA\"\t13179\t\"Evans County, GA\"\t13109\n\"Liberty County, GA\"\t13179\t\"Liberty County, GA\"\t13179\n\"Liberty County, GA\"\t13179\t\"Long County, GA\"\t13183\n\"Liberty County, GA\"\t13179\t\"McIntosh County, GA\"\t13191\n\"Liberty County, GA\"\t13179\t\"Tattnall County, GA\"\t13267\n\"Lincoln County, GA\"\t13181\t\"Columbia County, GA\"\t13073\n\"Lincoln County, GA\"\t13181\t\"Elbert County, GA\"\t13105\n\"Lincoln County, GA\"\t13181\t\"Lincoln County, GA\"\t13181\n\"Lincoln County, GA\"\t13181\t\"McDuffie County, GA\"\t13189\n\"Lincoln County, GA\"\t13181\t\"Wilkes County, GA\"\t13317\n\"Lincoln County, GA\"\t13181\t\"McCormick County, SC\"\t45065\n\"Long County, GA\"\t13183\t\"Liberty County, GA\"\t13179\n\"Long County, GA\"\t13183\t\"Long County, GA\"\t13183\n\"Long County, GA\"\t13183\t\"McIntosh County, GA\"\t13191\n\"Long County, GA\"\t13183\t\"Tattnall County, GA\"\t13267\n\"Long County, GA\"\t13183\t\"Wayne County, GA\"\t13305\n\"Lowndes County, GA\"\t13185\t\"Hamilton County, FL\"\t12047\n\"Lowndes County, GA\"\t13185\t\"Madison County, FL\"\t12079\n\"Lowndes County, GA\"\t13185\t\"Berrien County, GA\"\t13019\n\"Lowndes County, GA\"\t13185\t\"Brooks County, GA\"\t13027\n\"Lowndes County, GA\"\t13185\t\"Cook County, GA\"\t13075\n\"Lowndes County, 
